vi "test_AllCodeSourceOnly.vi"() -> (3 "Pass?":bool)   [LabVIEW 2019, in "Tests.General.lvlib"]
uses:
  Tests.General.lvlib
panel:
  out "Failed results":path[](array[path])
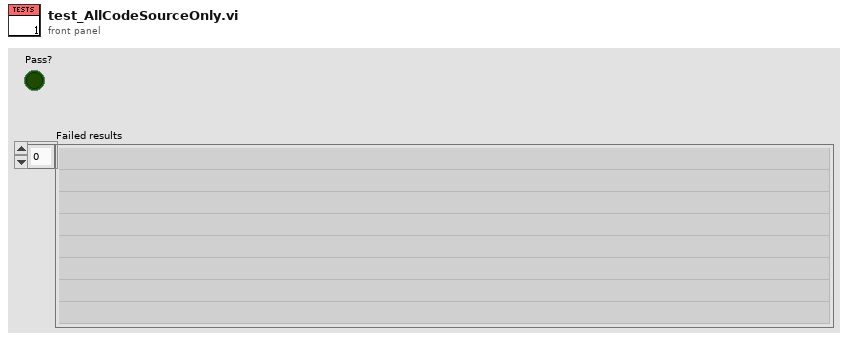
[diagram p1: front panel]
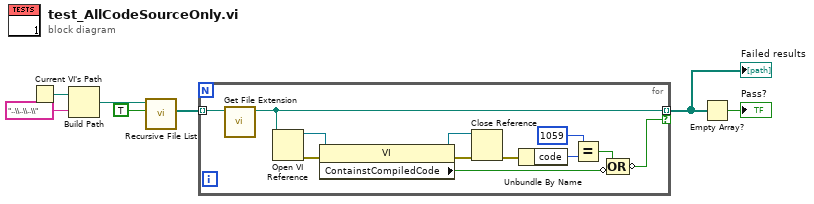
[diagram p0: block diagram]
diagram:
  n1 = Current VI's Path() -> (path=w7:path)
  n2 = Build Path(base path=w7, name or relative path="..\\..\\..\\") -> (appended path=w5:path)
  n3 = call <vilib>:"Recursive File List.vi"("Treat LLBs as Folders?"=TRUE, "Folder Path"=w5) -> ("All Files in Dir"=w3:path[])  [unwired: 5 in, 4 out]
  n4 = for {
    tunnel: w3 -> [w19] mode=indexing
    tunnel: [w11] -> w2 mode=indexing if=w17
    n5 = call <vilib>:"Get File Extension.vi"("file"=w19) -> ("dup file"=w11:path)  [unwired: 6 in, 4 out]
    n6 = Open VI Reference(vi path=w11) -> (vi reference=w14:refnum<vi>, error out=w13:errorcluster)  [unwired: 5 in]
    n7 = property class="VI"(reference=w14, error in=w13) -> (reference out=w9:refnum<vi>, error out=w10:errorcluster, "ContainstCompiledCode"=w12:bool)
    n8 = Close Reference(reference=w9, error in (no error)=w10) -> (error out=w8:errorcluster)
    n9 = Unbundle By Name(w8) -> ("code"=w16:i32)
    n10 = Equal?(x=1059 ("code"), y=w16) -> (x = y?=w18:bool)
    n11 = Compound Arithmetic op=OR(w18, invert w12) -> (invert w17:bool)
  }
  "Failed results" <- w2
  n12 = Empty Array?(array=w2) -> (empty?=→"Pass?":bool)
